vi "XNET Reflective Memory RT Driver VI.vi"(7 "Operation":T1, 11 "Device Reference in":T2 format="%.0x") -> (0 "Error Code":i32)   [LabVIEW 2010, in "XNET Reflective Memory Custom Device.lvlib"]
uses:
  XNET Reflective Memory Custom Device.lvlib
  <vilib>/NI Veristand/Custom Device API/Custom Device Item Ref.ctl
  <vilib>/NI Veristand/Custom Device API/Hardware Interface Driver VI Operation.ctl
  RT DATA.ctl
  Single Category.ctl
  BeforeAfter.ctl
  <vilib>/NI Veristand/Custom Device API/Data Reference.ctl
  Global.vi
  <vilib>/NI VeriStand/Custom Device API/Get Item Property (Boolean).vi
  <vilib>/NI VeriStand/Custom Device API/Get Item Property (U32).vi
  <vilib>/xnet/xnet.llb/XNET Write (Signal Single-point).vi
  <vilib>/xnet/xnet.llb/XNET Read (Signal Single-point).vi
  <vilib>/NI Veristand/Custom Device API/Custom Device API.lvlib
  Program Files/National Instruments/LabVIEW 2010/resource/objmgr/xnet.rc
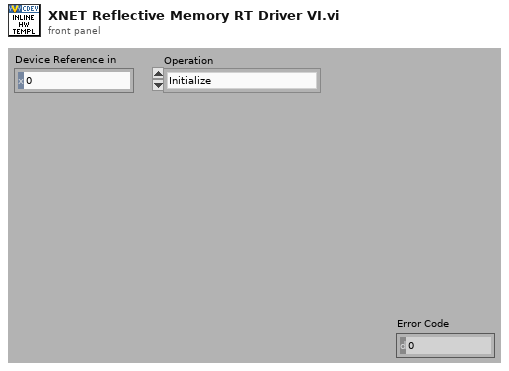
[diagram p1: front panel]
types:
  T1 = typedef "Custom Device API.lvlib/Hardware Interface Driver VI Operation.ctl" = enum16{"Initialize", "Start", "Read Data from HW", "Write Data to HW", "Close"}
  T2 = typedef "Custom Device API.lvlib/Custom Device Item Ref.ctl" = u64
  T3 = typedef "XNET Reflective Memory Custom Device.lvlib/RT DATA.ctl" = cluster{" Inputs":T4, "Outputs":T4, "Internal Iteration":i32, "Device Error":errorcluster}
  T4 = typedef "XNET Reflective Memory Custom Device.lvlib/Single Category.ctl" = cluster{"Vals":dbl[], "When":T5[], "Data Refs":T6[], "Session":refnum<k21>, "NIT Start":u32}
  T5 = typedef "XNET Reflective Memory Custom Device.lvlib/BeforeAfter.ctl" = enum16{"Before", "After"}
  T6 = typedef "Custom Device API.lvlib/Data Reference.ctl" = i32
  T7 = typedef "XNET Reflective Memory Custom Device.lvlib/Action.ctl" = enum16{"Before Write", "After Read", "After Write", "Before Read", "None"}
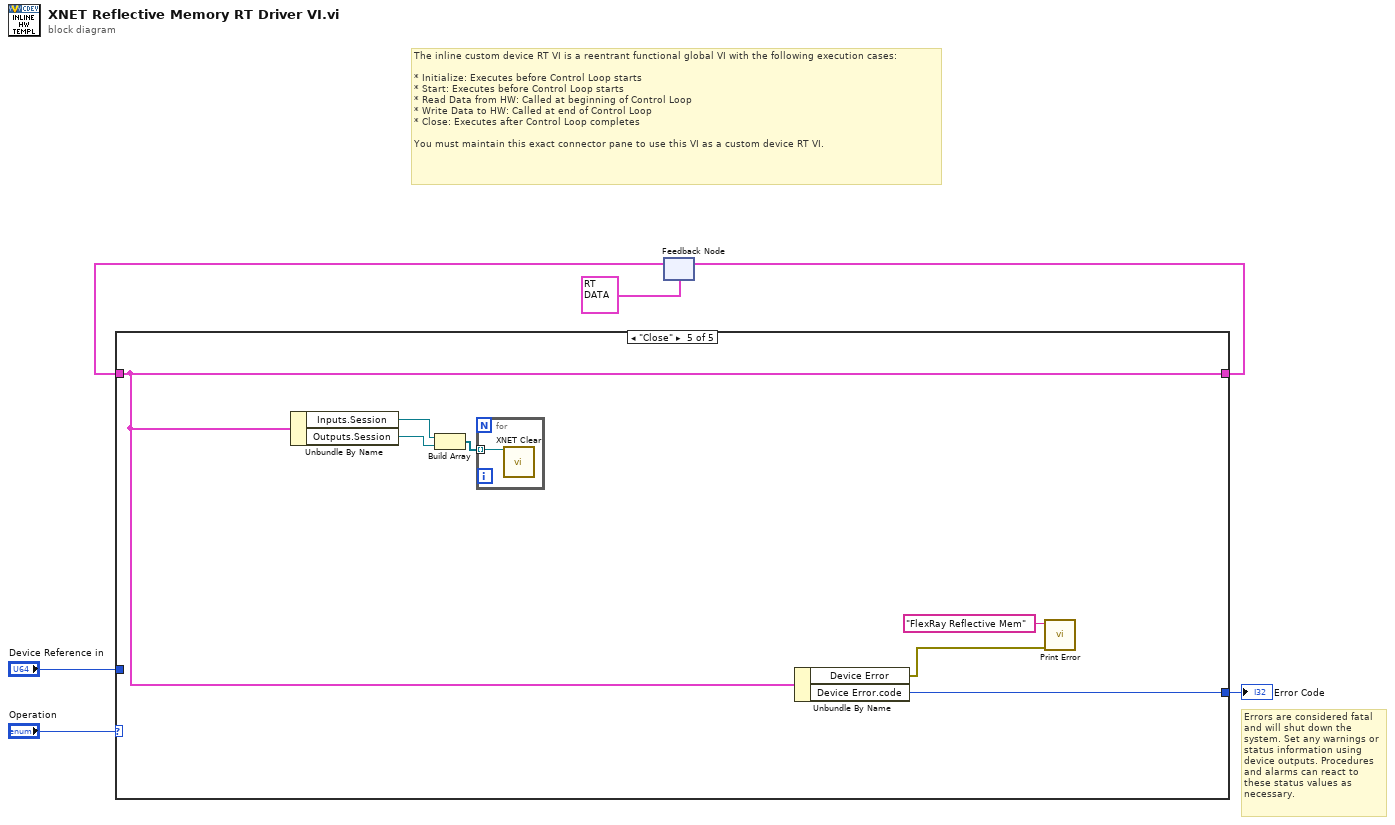
[diagram p0: block diagram]
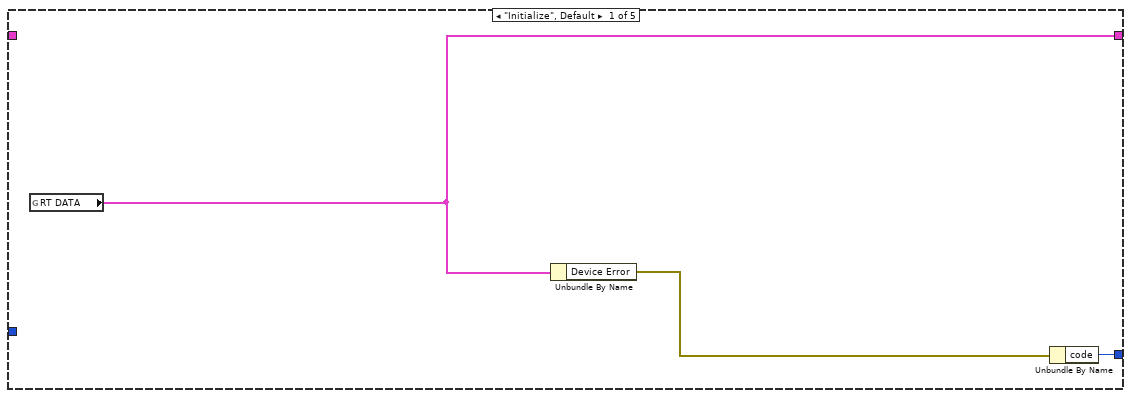
[diagram p2: hidden frame]
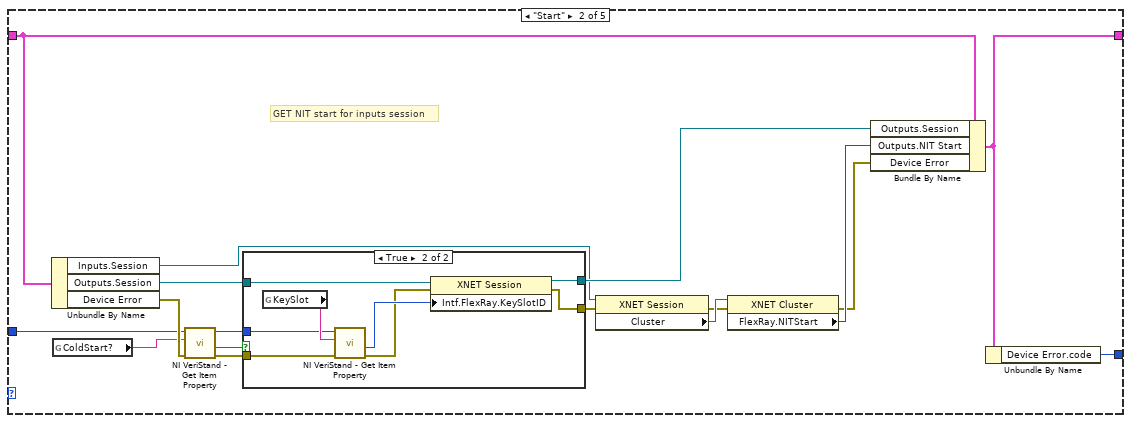
[diagram p3: hidden frame]
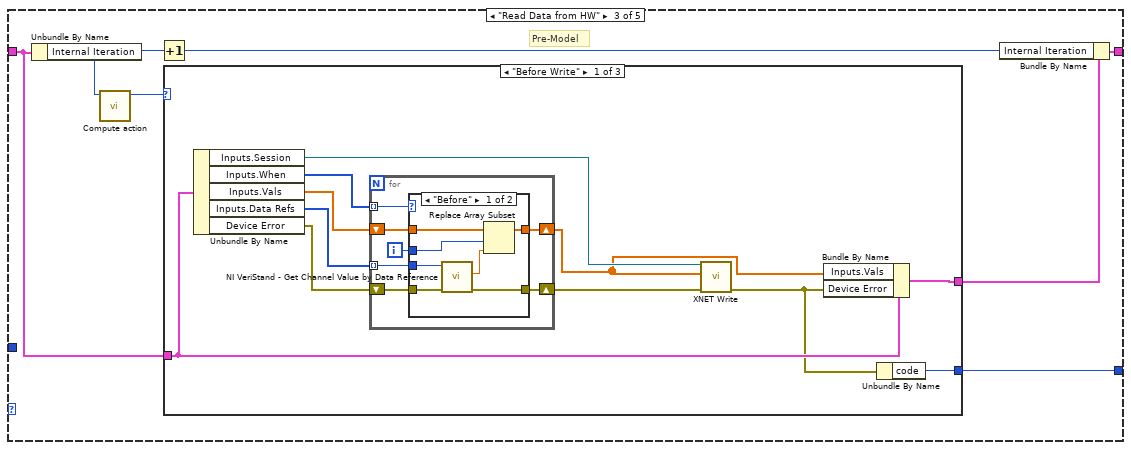
[diagram p5: hidden frame]
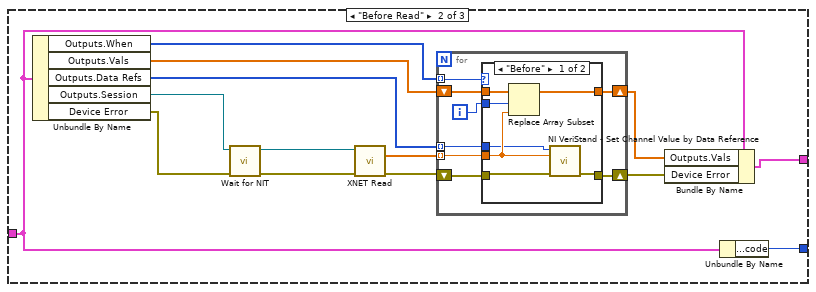
[diagram p7: hidden frame]
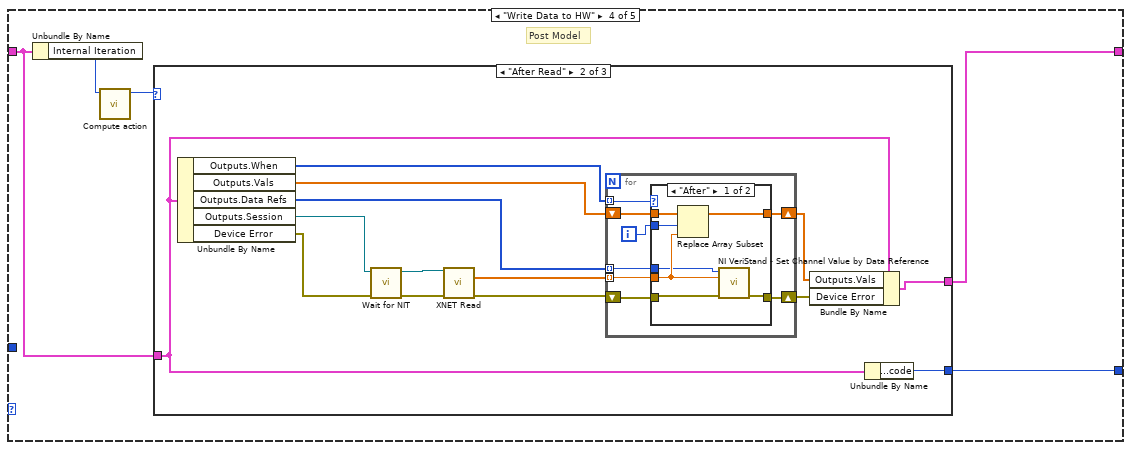
[diagram p10: hidden frame]
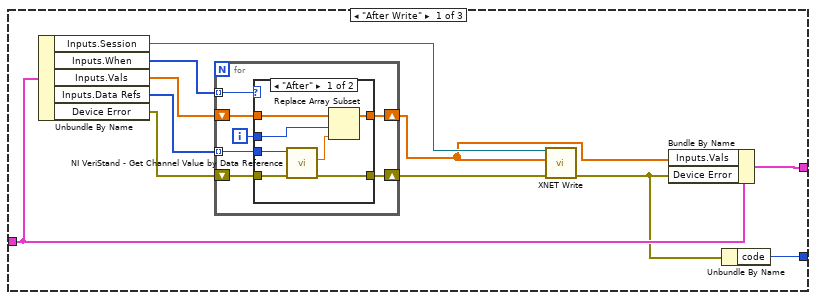
[diagram p11: hidden frame]
diagram:
  # "Errors are considered fatal and will shut down the system. Set any warnings or status information using device outputs. Procedures and alarms can react to these status values as necessary."
  # "The inline custom device RT VI is a reentrant functional global VI with the following execution cases:\n\n* Initialize: Executes before Control Loop starts\n* Start: Executes before Control Loop starts\n* Read Data from HW: Called at beginning of Control Loop\n* Write Data to HW: Called at end of Control Loop\n* Close: Executes after Control Loop completes\n\nYou must maintain this exact connector pane to use this VI as a custom device RT VI."
  n1 = feedback #1(T3 {" Inputs"={"Vals"=[], "When"=[], "Data Refs"=[], "Session"="", "NIT Start"=0}, "Outputs"={"Vals"=[], "When"=[], "Data Refs"=[], "Session"="", "NIT Start"=0}, "Internal Iteration"=0, "Device Error"={"status"=FALSE, "code"=0, "source"=""}} ("cluster")) -> (w4:T3)
  n2 = case shown="\"Close\"" "Operation" {
    tunnel: [w7 w24 w40 w106 w170] -> w5
    tunnel: w4 -> [_ w25 w42 w104 w170]
    tunnel: "Device Reference in" -> [_ w22 _ _ _]
    tunnel: [w9 w26 w43 w105 w173] -> w2
    frame "Initialize", Default {
      n3 = global read "Global.vi" "RT DATA"() -> (w7:T3)
      n4 = Unbundle By Name(w7) -> ("Device Error"=w8:errorcluster)
      n5 = Unbundle By Name(w8) -> ("code"=w9:i32)
    }
    frame "Start" {
      # "GET NIT start for inputs session"
      n6 = Unbundle By Name(w25) -> ("Inputs.Session"=w12:refnum<k21>, "Outputs.Session"=w17:refnum<k21>, "Device Error"=w23:errorcluster)
      n7 = global read "Global.vi" "ColdStart?"() -> (w21:string)
      n8 = call-poly <vilib>:"NI VeriStand - Get Item Property.vi"("error in (no error)"=w23, "Property Name"=w21, "Item Ref in"=w22) -> ("error out"=w19:errorcluster, "Value"=w20:bool, "Item Ref out"=w18:T2)  [unwired: 5 in, 1 out]
      n9 = case shown="True" w20 {
        tunnel: w19 -> [w28 w36]
        tunnel: w18 -> [_ w34]
        tunnel: w17 -> [w27 w33]
        tunnel: [w27 w32] -> w16
        tunnel: [w28 w29] -> w15
        frame False {
        }
        frame True {
          n10 = global read "Global.vi" "KeySlot"() -> (w35:string)
          n11 = call-poly <vilib>:"NI VeriStand - Get Item Property.vi"("error in (no error)"=w36, "Property Name"=w35, "Item Ref in"=w34) -> ("error out"=w30:errorcluster, "Value"=w31:u32)  [unwired: 5 in, 2 out]
          n12 = property class="XNET Session"(reference=w33, error in=w30, "Intf.FlexRay.KeySlotID"=w31) -> (reference out=w32:refnum<k21>, error out=w29:errorcluster)
        }
      }
      n13 = property class="XNET Session"(reference=w12, error in=w15) -> (error out=w13:errorcluster, "Cluster"=w14:refnum<k21>)  [unwired: 1 out]
      n14 = property class="XNET Cluster"(reference=w14, error in=w13) -> (error out=w10:errorcluster, "FlexRay.NITStart"=w11:u32)  [unwired: 1 out]
      n15 = Bundle By Name(cluster=w25, "Outputs.Session"=w16, "Outputs.NIT Start"=w11, "Device Error"=w10) -> (w24:T3)
      n16 = Unbundle By Name(w24) -> ("Device Error.code"=w26:i32)
    }
    frame "Read Data from HW" {
      # "Pre-Model"
      n17 = Unbundle By Name(w42) -> ("Internal Iteration"=w38:i32)
      n18 = call "Compute action.vi"("Iteration"=w38) -> ("Action"=w37:T7)  [unwired: 10 in]
      n19 = Increment(x=w38) -> (x+1=w39:i32)
      n20 = case shown="\"Before Write\"" w37 {
        tunnel: [w50 w84 _] -> w43
        tunnel: w42 -> [w54 w78 w102]
        tunnel: [w53 w77 w102] -> w41
        frame "Before Write" {
          n21 = Unbundle By Name(w54) -> ("Inputs.Session"=w52:refnum<k21>, "Inputs.When"=w48:T5[], "Inputs.Vals"=w46:dbl[], "Inputs.Data Refs"=w47:T6[], "Device Error"=w49:errorcluster)
          n22 = for {
            shift-right: [w58] -> w44
            shift-left: w49 -> [w60]
            tunnel: w48 -> [w61] mode=indexing
            tunnel: w47 -> [w59] mode=indexing
            shift-right: [w55] -> w45
            shift-left: w46 -> [w56]
            i -> [w57]
            n23 = case shown="\"Before\"" w61 {
              tunnel: w60 -> [w68 w70]
              tunnel: w59 -> [w67 _]
              tunnel: [w65 w70] -> w58
              tunnel: w57 -> [w64 _]
              tunnel: w56 -> [w63 w69]
              tunnel: [w62 w69] -> w55
              frame "Before" {
                n24 = call <vilib>:"NI VeriStand - Get Channel Value by Data Reference.vi"("error in (no error)"=w68, "Data Reference in"=w67) -> ("error out"=w65:errorcluster, "Value"=w66:dbl)  [unwired: 8 in]
                n25 = Replace Array Subset(array=w63, new element=w66, index=w64) -> (w62:dbl[])
              }
              frame Default {
              }
            }
          }
          n26 = call-poly <vilib>:"XNET Write.vi"("session in"=w52, "data"=w45, "error in (no error)"=w44) -> ("error out"=w51:errorcluster)  [unwired: 11 in, 1 out]
          n27 = Bundle By Name(cluster=w54, "Inputs.Vals"=w45, "Device Error"=w51) -> (w53:T3)
          n28 = Unbundle By Name(w51) -> ("code"=w50:i32)
        }
        frame "Before Read" {
          n29 = Unbundle By Name(w78) -> ("Outputs.When"=w83:T5[], "Outputs.Vals"=w82:dbl[], "Outputs.Data Refs"=w80:T6[], "Outputs.Session"=w72:refnum<k21>, "Device Error"=w71:errorcluster)
          n30 = call "Wait for NIT.vi"("Error"=w71, "session in"=w72) -> ("Error out"=w74:errorcluster, "session out"=w73:refnum<k21>)  [unwired: 8 in]
          n31 = call-poly <vilib>:"XNET Read.vi"("session in"=w73, "error in (no error)"=w74) -> ("data"=w75:dbl[], "error out"=w81:errorcluster)  [unwired: 11 in, 1 out]
          n32 = for {
            shift-right: [w91] -> w79
            shift-left: w81 -> [w92]
            shift-right: [w88] -> w76
            shift-left: w82 -> [w89]
            tunnel: w83 -> [w87] mode=indexing
            tunnel: w75 -> [w86] mode=indexing
            tunnel: w80 -> [w85] mode=indexing
            i -> [w90]
            n33 = case shown="\"Before\"" w87 {
              tunnel: w92 -> [w96 w101]
              tunnel: [w95 w101] -> w91
              tunnel: w90 -> [w99 _]
              tunnel: w89 -> [w98 w100]
              tunnel: [w97 w100] -> w88
              tunnel: w86 -> [w94 _]
              tunnel: w85 -> [w93 _]
              frame "Before" {
                n34 = Replace Array Subset(array=w98, new element=w94, index=w99) -> (w97:dbl[])
                n35 = call <vilib>:"NI VeriStand - Set Channel Value by Data Reference.vi"("error in (no error)"=w96, "Value"=w94, "Data Reference in"=w93) -> ("error out"=w95:errorcluster)  [unwired: 8 in]
              }
              frame Default {
              }
            }
          }
          n36 = Bundle By Name(cluster=w78, "Outputs.Vals"=w76, "Device Error"=w79) -> (w77:T3)
          n37 = Unbundle By Name(w78) -> ("Device Error.code"=w84:i32)
        }
        frame Default {
        }
      }
      n38 = Bundle By Name(cluster=w41, "Internal Iteration"=w39) -> (w40:T3)
    }
    frame "Write Data to HW" {
      # "Post Model"
      n39 = Unbundle By Name(w104) -> ("Internal Iteration"=w107:i32)
      n40 = call "Compute action.vi"("Iteration"=w107) -> ("Action"=w103:T7)  [unwired: 10 in]
      n41 = case shown="\"After Read\"" w103 {
        tunnel: [w114 w148 _] -> w105
        tunnel: w104 -> [w118 w141 w166]
        tunnel: [w117 w140 w166] -> w106
        frame "After Write" {
          n42 = Unbundle By Name(w118) -> ("Inputs.Session"=w116:refnum<k21>, "Inputs.When"=w112:T5[], "Inputs.Vals"=w110:dbl[], "Inputs.Data Refs"=w111:T6[], "Device Error"=w113:errorcluster)
          n43 = for {
            shift-right: [w122] -> w109
            shift-left: w113 -> [w124]
            tunnel: w112 -> [w125] mode=indexing
            tunnel: w111 -> [w123] mode=indexing
            shift-right: [w119] -> w108
            shift-left: w110 -> [w120]
            i -> [w121]
            n44 = case shown="\"After\"" w125 {
              tunnel: w124 -> [w132 w134]
              tunnel: w123 -> [w131 _]
              tunnel: [w129 w134] -> w122
              tunnel: w121 -> [w128 _]
              tunnel: w120 -> [w127 w133]
              tunnel: [w126 w133] -> w119
              frame "After" {
                n45 = call <vilib>:"NI VeriStand - Get Channel Value by Data Reference.vi"("error in (no error)"=w132, "Data Reference in"=w131) -> ("error out"=w129:errorcluster, "Value"=w130:dbl)  [unwired: 8 in]
                n46 = Replace Array Subset(array=w127, new element=w130, index=w128) -> (w126:dbl[])
              }
              frame Default {
              }
            }
          }
          n47 = call-poly <vilib>:"XNET Write.vi"("session in"=w116, "data"=w108, "error in (no error)"=w109) -> ("error out"=w115:errorcluster)  [unwired: 11 in, 1 out]
          n48 = Bundle By Name(cluster=w118, "Inputs.Vals"=w108, "Device Error"=w115) -> (w117:T3)
          n49 = Unbundle By Name(w115) -> ("code"=w114:i32)
        }
        frame "After Read" {
          n50 = Unbundle By Name(w141) -> ("Outputs.When"=w147:T5[], "Outputs.Vals"=w146:dbl[], "Outputs.Data Refs"=w143:T6[], "Outputs.Session"=w136:refnum<k21>, "Device Error"=w135:errorcluster)
          n51 = call "Wait for NIT.vi"("Error"=w135, "session in"=w136) -> ("Error out"=w138:errorcluster, "session out"=w137:refnum<k21>)  [unwired: 8 in]
          n52 = call-poly <vilib>:"XNET Read.vi"("session in"=w137, "error in (no error)"=w138) -> ("data"=w144:dbl[], "error out"=w145:errorcluster)  [unwired: 11 in, 1 out]
          n53 = for {
            shift-right: [w155] -> w142
            shift-left: w145 -> [w156]
            shift-right: [w152] -> w139
            shift-left: w146 -> [w153]
            tunnel: w147 -> [w151] mode=indexing
            tunnel: w144 -> [w150] mode=indexing
            tunnel: w143 -> [w149] mode=indexing
            i -> [w154]
            n54 = case shown="\"After\"" w151 {
              tunnel: w156 -> [w160 w165]
              tunnel: [w159 w165] -> w155
              tunnel: w154 -> [w163 _]
              tunnel: w153 -> [w162 w164]
              tunnel: [w161 w164] -> w152
              tunnel: w150 -> [w158 _]
              tunnel: w149 -> [w157 _]
              frame "After" {
                n55 = Replace Array Subset(array=w162, new element=w158, index=w163) -> (w161:dbl[])
                n56 = call <vilib>:"NI VeriStand - Set Channel Value by Data Reference.vi"("error in (no error)"=w160, "Value"=w158, "Data Reference in"=w157) -> ("error out"=w159:errorcluster)  [unwired: 8 in]
              }
              frame Default {
              }
            }
          }
          n57 = Bundle By Name(cluster=w141, "Outputs.Vals"=w139, "Device Error"=w142) -> (w140:T3)
          n58 = Unbundle By Name(w141) -> ("Device Error.code"=w148:i32)
        }
        frame Default {
        }
      }
    }
    frame "Close" {
      n59 = Unbundle By Name(w170) -> ("Inputs.Session"=w169:refnum<k21>, "Outputs.Session"=w172:refnum<k21>)
      n60 = Build Array(w169, w172) -> (w171:refnum<k21>[])
      n61 = for {
        tunnel: w171 -> [w174] mode=indexing
        n62 = call <vilib>:"XNET Clear.vi"("session in"=w174) -> ()  [unwired: 14 in, 1 out]
      }
      n63 = Unbundle By Name(w170) -> ("Device Error"=w167:errorcluster, "Device Error.code"=w173:i32)
      n64 = call "Print Error.vi"("error out"=w167, "Your code's public name"="FlexRay Reflective Mem") -> ()  [unwired: 9 in]
    }
  }
  "Error Code" <- w2
  n65 = feedback-in #1(w5) -> ()
